vi "Read Mutation.vi"(8 "error in (no error)":errorcluster, 11 "TSP Class in":refnum<class "TSP Class.lvclass">) -> (0 "error out":errorcluster, 2 "Mutation":T1, 3 "TSP Class out":refnum<class "TSP Class.lvclass">)   [LabVIEW 2015, in "TSP Library.lvlib" / "TSP Class.lvclass"]
uses:
  TSP Class.lvclass
  TypeDef/Mutation.ctl
  TSP Class.lvclass/TSP Class.ctl
  TSP Library.lvlib
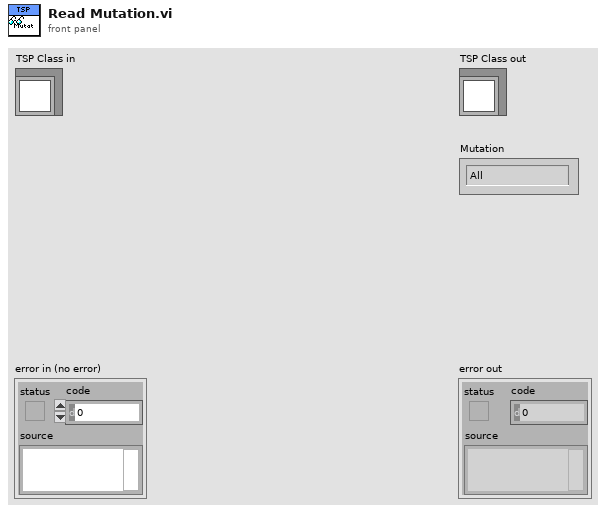
[diagram p1: front panel]
types:
  T1 = typedef "TSP Library.lvlib/Mutation.ctl" = enum16{"All", "Roulette"}
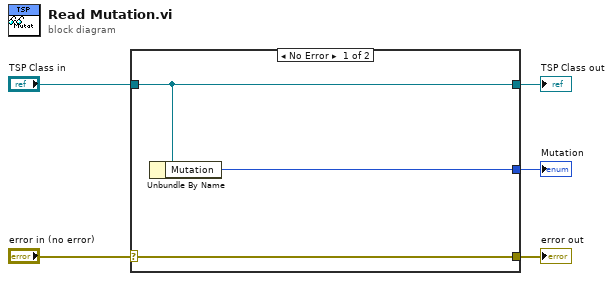
[diagram p0: block diagram]
diagram:
  n1 = case shown="No Error" "error in (no error)" {
    selector: "error in (no error)" -> [w8 w9]
    tunnel: [w8 w9] -> w4
    tunnel: [w7 w10] -> w2
    tunnel: "TSP Class in" -> [w7 w10]
    tunnel: [w6 _] -> w1
    frame No Error {
      n2 = Unbundle By Name(w7) -> ("Mutation"=w6:T1)
    }
    frame Error {
    }
  }
  "error out" <- w4
  "TSP Class out" <- w2
  "Mutation" <- w1
